vi "to Array.vi"(8 "error in (no error)":errorcluster, 11 "Output Value in":refnum<class "Output Value.lvclass">) -> (0 "error out":errorcluster, 2 "Output values":dbl[](array[numeric]), 3 "Output Value out":refnum<class "Output Value.lvclass">)   [LabVIEW 2019, in "Output Value.lvclass"]
uses:
  Output Value.lvclass
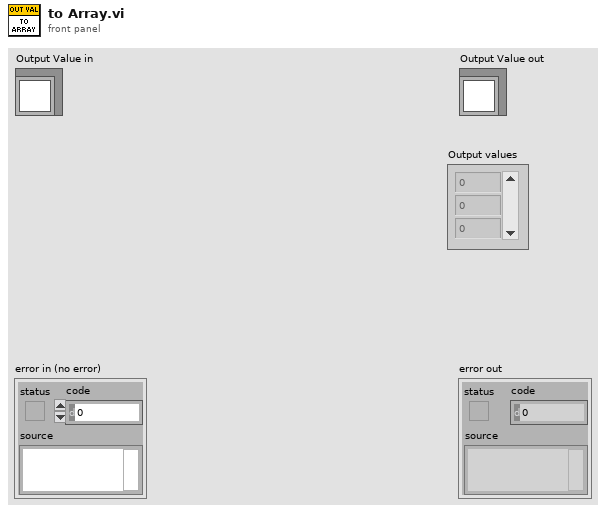
[diagram p1: front panel]
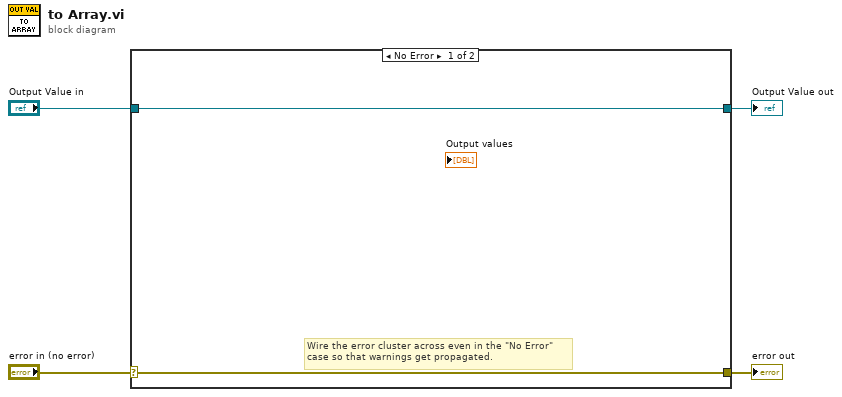
[diagram p0: block diagram]
diagram:
  n1 = case shown="No Error" "error in (no error)" {
    selector: "error in (no error)" -> [w5 w8]
    tunnel: [w5 w8] -> w3
    tunnel: [w6 w7] -> w1
    tunnel: "Output Value in" -> [w6 w7]
    frame No Error {
      # "Wire the error cluster across even in the \"No Error\"\ncase so that warnings get propagated."
    }
    frame Error {
    }
  }
  "error out" <- w3
  "Output Value out" <- w1
